vi "ESP301 MotorEn.vi"(6 "Set":bool, 8 "error in":errorcluster, 9 "Axis":i8(ring)=1 items=["Axis 1"=1, "Axis 2"=2, "Axis 3"=3], 10 "MotorEn":bool, 11 "VISA Rsrc":refnum<visa-resource-name>="GPIB0::7::INSTR") -> (0 "error out":errorcluster, 3 "MotorEnOut":bool)   [LabVIEW 2019]
uses:
  <userlib>/ESP300/ESP300 GotoState.ctl
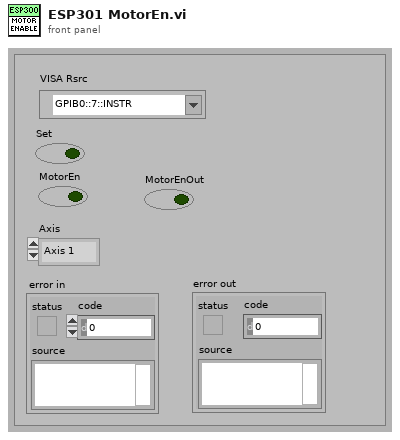
[diagram p1: front panel]
types:
  T1 = typedef "ESP300 GotoState.ctl" = enum16{"send command", "read position", "check status", "end"}
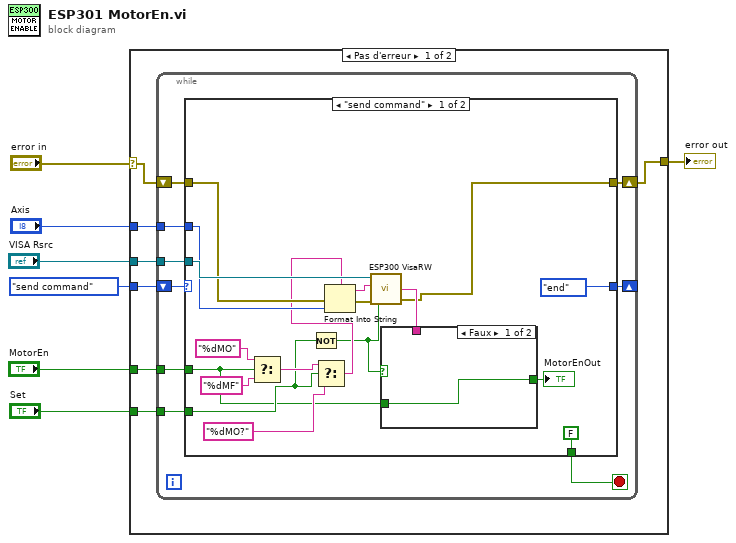
[diagram p0: block diagram]
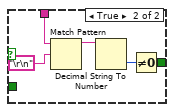
[diagram p2: hidden frame]
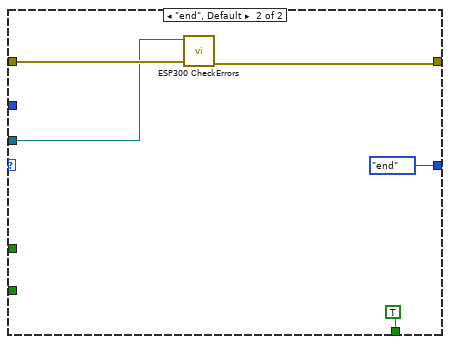
[diagram p3: hidden frame]
diagram:
  n1 = case shown="Pas d'erreur" "error in" {
    selector: "error in" -> [w12 w53]
    tunnel: "Axis" -> [w14 _]
    tunnel: [w11 w53] -> w5
    tunnel: ESP300_GotoState."send command" ("Énum") -> [w13 _]
    tunnel: "VISA Rsrc" -> [w10 _]
    tunnel: "MotorEn" -> [w9 _]
    tunnel: "Set" -> [w8 _]
    frame No Error {
      n2 = while {
        tunnel: w14 -> [w23]
        shift-right: [w19] -> w11
        shift-left: w12 -> [w21]
        tunnel: w10 -> [w20]
        shift-right: [w17] -> _
        shift-left: w13 -> [w22]
        tunnel: w9 -> [w16]
        tunnel: w8 -> [w15]
        stop <- w18 stop-if-true
        n3 = case shown="\"send command\"" w22 {
          tunnel: w23 -> [w40 _]
          tunnel: w21 -> [w39 w50]
          tunnel: w20 -> [w41 w48]
          tunnel: [w34 w49] -> w19
          tunnel: [FALSE TRUE] -> w18
          tunnel: [ESP300_GotoState."end" ("Énum") ESP300_GotoState."end" ("Énum")] -> w17
          tunnel: w16 -> [w24 _]
          tunnel: w15 -> [w26 _]
          frame "send command" {
            n4 = Select(t="%dMO" ("format string"), s=w24, f="%dMF" ("format string")) -> (s? t:f=w30:string)
            n5 = Not(x=w26) -> (.not. x?=w25:bool)
            n6 = Select(t=w30, s=w26, f="%dMO?" ("format string")) -> (s? t:f=w28:string)
            n7 = Format Into String(format string=w28, error in=w39, w40) -> (resulting string=w29:string, error out=w38:errorcluster)  [unwired: 1 in]
            n8 = call <userlib>:"ESP300 VisaRW.vi"("Lecture?(T)"=w25, "error in (no error)"=w38, "ChaineCom"=w29, "VISA Rsrc"=w41) -> ("error out"=w34:errorcluster, "ChaineRep"=w35:string)  [unwired: 3 in, 2 out]
            n9 = case shown="Faux" w25 {
              tunnel: w35 -> [_ w46]
              tunnel: [w42 w43] -> w33
              tunnel: w24 -> [w42 _]
              frame False {
              }
              frame True {
                n10 = Match Pattern(string=w46, regular expression="\r\n") -> (before substring=w45:string)  [unwired: 1 in, 3 out]
                n11 = Decimal String To Number(string=w45) -> (number=w44:i32)  [unwired: 2 in, 1 out]
                n12 = Not Equal To 0?(x=w44) -> (x != 0?=w43:bool)
              }
            }
            "MotorEnOut" <- w33
          }
          frame "end", Default {
            n13 = call <userlib>:"ESP300 CheckErrors.vi"("error in (no error)"=w50, "Ressource VISA In"=w48) -> ("error out"=w49:errorcluster)  [unwired: 4 in, 3 out]
          }
        }
      }
    }
    frame Error {
    }
  }
  "error out" <- w5
